vi "FinalProject.vi"() -> ()   [LabVIEW 2021]
uses:
  <vilib>/Utility/file.llb/Write Delimited Spreadsheet (DBL).vi
  <vilib>/Utility/file.llb/Write Delimited Spreadsheet (string).vi
  <vilib>/express/express arith-compare/Formula/XNode/ExpressFormulaBlockNode.xnode
  <vilib>/Analysis/NI_AALBase.lvlib
panel:
  in  "File Path":path
  in  "format (%.3f)":string="%.3f"
  in  "stop":bool
  out "Time [s]":dbl
  out "Waveform Graph":waveform(dbl)(graph)
  out "Power Standard Deviation [W]":dbl format="%0.5f"
  out "Power Average [W]":dbl format="%0.5f"
  out "Voltage Standard Deviation [V]":dbl format="%0.5f"
  out "Voltage Average. [V]":dbl format="%0.5f"
  in  "device name":tag="Dev1"
  in  "Number of Samples [-]":i32=100
  in  "Sampling Rate [Hz]":dbl=1000.0
  in  "Resistance [Ohms]":dbl
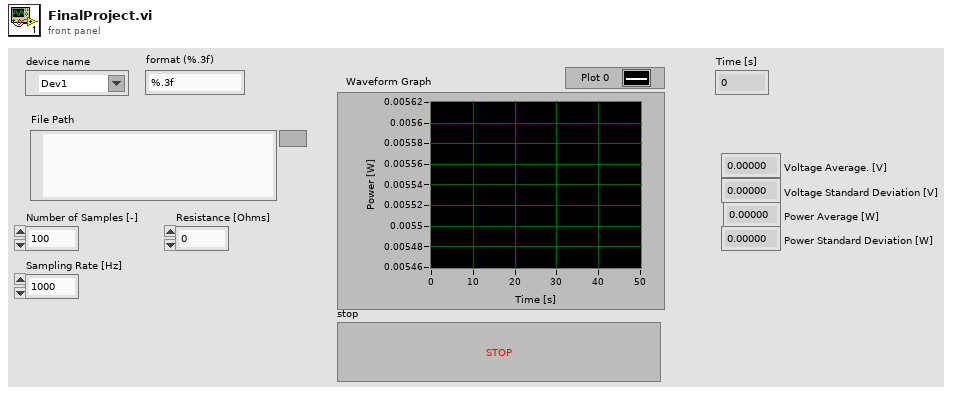
[diagram p1: front panel]
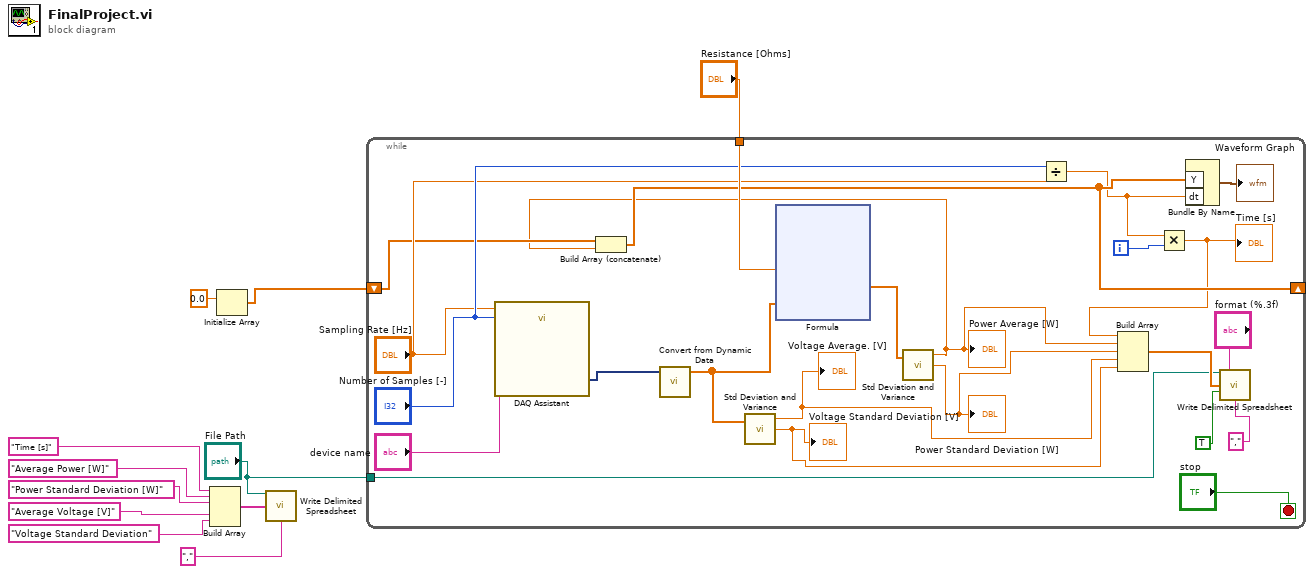
[diagram p0: block diagram]
diagram:
  n1 = Build Array("Time [s]", "Average Power [W]", "Power Standard Deviation [W]", "Average Voltage [V]", "Voltage Standard Deviation") -> (w4:string[])
  n2 = Initialize Array(0.0 ("element")) -> (w9:dbl[])  [unwired: 1 in]
  n3 = call-poly <vilib>:"Write Delimited Spreadsheet.vi"("file path (dialog if empty)"="File Path", "1D data"=w4, "delimiter (\\t)"=",") -> ()  [unwired: 11 in, 2 out]
  n4 = while {
    tunnel: "Resistance [Ohms]" -> [w34]
    shift-right: [w25] -> _
    shift-left: w9 -> [w26]
    tunnel: "File Path" -> [w12]
    i -> [w23]
    stop <- "stop" stop-if-true
    n5 = call "DAQ Assistant"("rate"="Sampling Rate [Hz]", "number of samples"="Number of Samples [-]", "device name"="device name") -> ("data"=w33:dynamicdata)  [unwired: 14 in, 2 out]
    n6 = call "Convert from Dynamic Data"("Dynamic Data Type"=w33) -> ("Array"=w31:dbl[])  [unwired: 3 in]
    n7 = call <vilib>:"Std Deviation and Variance.vi"("X"=w31) -> ("mean"=w16:dbl, "standard deviation"=w15:dbl)  [unwired: 1 in, 1 out]
    "Voltage Average. [V]" <- w16
    "Voltage Standard Deviation [V]" <- w15
    n8 = xnode "Formula"("R"=w34, "V"=w31) -> ("Result"=w30:dbl[])  [unwired: 1 in, 1 out]
    n9 = call <vilib>:"Std Deviation and Variance.vi"("X"=w30) -> ("mean"=w18:dbl, "standard deviation"=w17:dbl)  [unwired: 1 in, 1 out]
    "Power Average [W]" <- w18
    "Power Standard Deviation [W]" <- w17
    n10 = Build Array (concatenate)(w26, w18) -> (w25:dbl[])
    n11 = Divide(x="Number of Samples [-]", y="Sampling Rate [Hz]") -> (x/y=w24:dbl)
    n12 = Multiply(x=w24, y=w23) -> (x*y=w14:dbl)
    "Time [s]" <- w14
    n13 = Build Array(w14, w18, w17, w16, w15) -> (w13:dbl[])
    n14 = Bundle By Name("Y"=w25, "dt"=w24) -> (→"Waveform Graph":waveform(dbl))  [unwired: 1 in]
    n15 = call-poly <vilib>:"Write Delimited Spreadsheet.vi"("file path (dialog if empty)"=w12, "format (%.3f)"="format (%.3f)", "1D data"=w13, "append to file? (new file:F)"=TRUE, "delimiter (\\t)"=",") -> ()  [unwired: 9 in, 2 out]
  }
